vi "Post_Pro_Results_Hierarchy.vi"() -> ()   [LabVIEW 2010]
uses:
  Anemometry Sub Vis/Controls/Setup.ctl
panel:
  out "Error":string
  out "Unfound Files":i32
  out "Processed Files":i32
  in  "Select Plug Ins":bool
  out "Results files Processed":i32(slide) scale=0.0..1.0
  in  "stop":bool
  out "Files To Process":path[](array[path])
  in  "Post processed Results folder":path
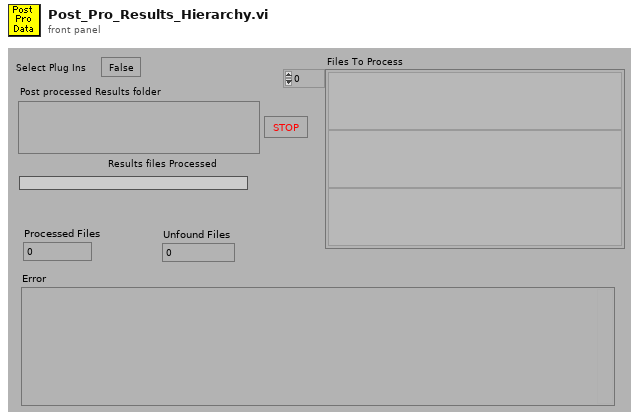
[diagram p1: front panel]
types:
  T1 = typedef "Setup.ctl" = enum16{"Run Program", "Show Setup", "Save Current Setup", "Setup Front Panel"}
  T2 = enum32{"existing file", "new file", "new or existing file", "existing dir", "new dir", "new or existing dir", "existing file (use LLBs)", "new file (use LLBs)", "new or existing file (use LLBs)", "new or existing file or directory (use LLBs)"}
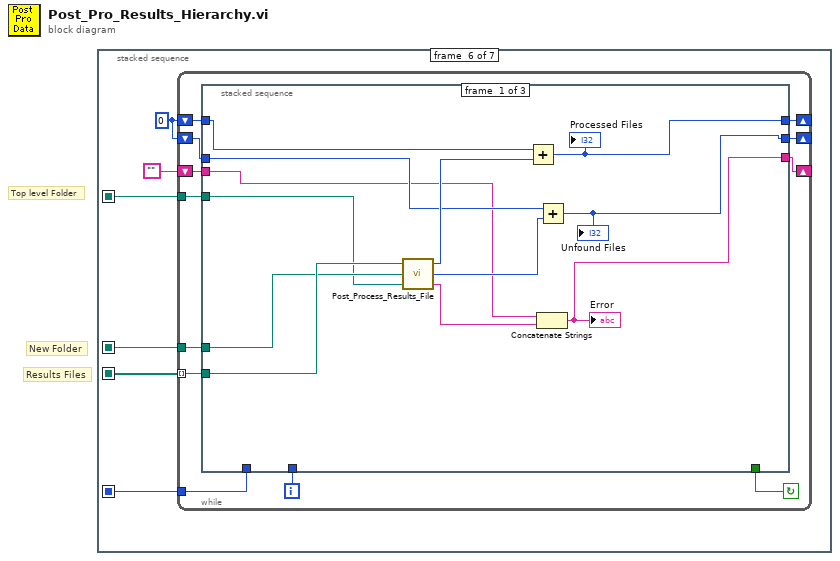
[diagram p0: block diagram]
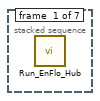
[diagram p2: hidden frame]
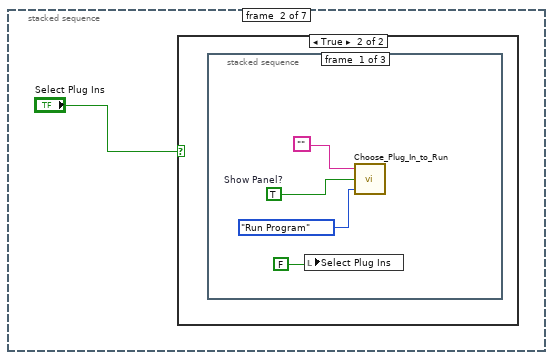
[diagram p3: hidden frame]
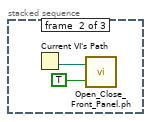
[diagram p5: hidden frame]
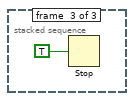
[diagram p6: hidden frame]
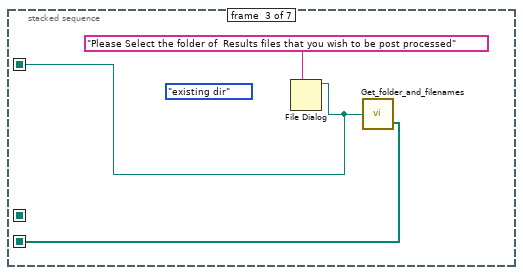
[diagram p7: hidden frame]
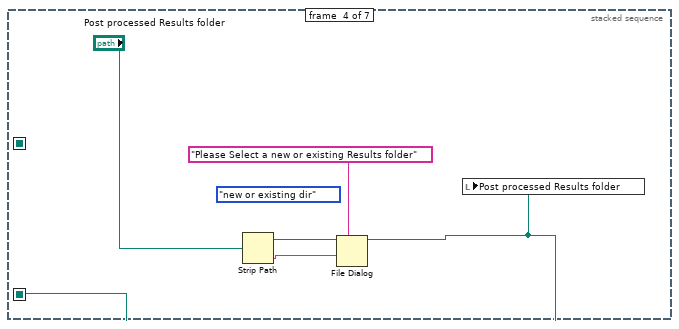
[diagram p8: hidden frame]
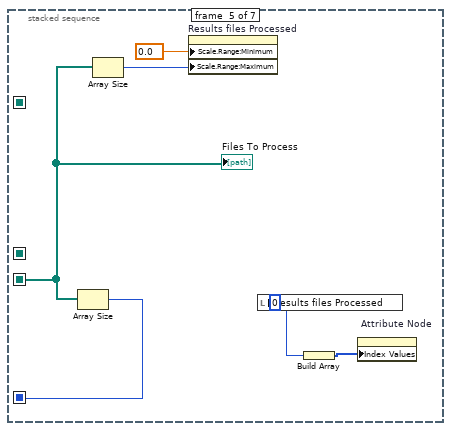
[diagram p9: hidden frame]
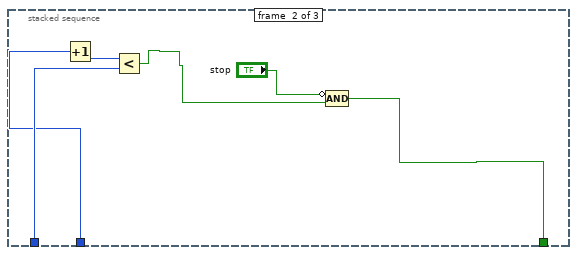
[diagram p10: hidden frame]
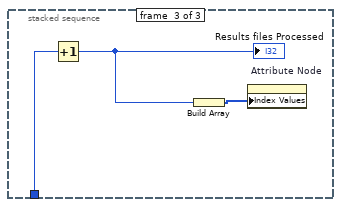
[diagram p11: hidden frame]
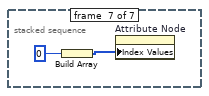
[diagram p12: hidden frame]
diagram:
  # "Top level Folder"
  # "New Folder"
  # "Results Files"
  n1 = stacked-sequence {
    seq-local: [_ _ w9 _ _ _ _] -> [_ _ _ _ _ w25 _]
    seq-local: [_ _ _ _ w22 _ _] -> [_ _ _ _ _ w28 _]
    seq-local: [_ _ _ w16 _ _ _] -> [_ _ _ _ _ w26 _]
    seq-local: [_ _ w10 _ _ _ _] -> [_ _ _ _ w17 w27 _]
    frame #0 {
      n2 = call "Run_EnFlo_Hub.vi"() -> ()  [unwired: 8 in]
    }
    frame #1 {
      n3 = case shown="True" "Select Plug Ins" {
        frame False {
        }
        frame True {
          n4 = stacked-sequence {
            frame #0 {
              w5 = TRUE  # Show Panel?
              n5 = local write "Select Plug Ins"(FALSE ("Select Local ADAM Channels")) -> ()
              n6 = call "Choose_Plug_In_to_Run.vi"("setup"=Setup."Run Program", "Show Panel?"=w5, "Setup String In"="") -> ()  [unwired: 1 in, 1 out]
            }
            frame #1 {
              n7 = Current VI's Path() -> (path=w7:path)
              n8 = call "Open_Close_Front_Panel.ph.vi"("Front Panel Window:Open"=TRUE, "VI path"=w7) -> ()  [unwired: 1 in, 1 out]
            }
            frame #2 {
              n9 = Stop(stop? (T)=TRUE) -> ()
            }
          }
        }
      }
    }
    frame #2 {
      (unwired) T2."existing dir" ("select mode (2)")
      n10 = File Dialog(7:"Please Select the folder of  Results files that you wish to be post processed" ("prompt")) -> (3:w9:path)  [unwired: 6 in, 3 out]
      n11 = call "Get_folder_and_filenames.vi"("file path (dialog if empty)"=w9) -> ("Files"=w10:path[])  [unwired: 1 out]
    }
    frame #3 {
      (unwired) T2."new or existing dir" ("select mode (2)")
      n12 = Strip Path(path="Post processed Results folder") -> (stripped path=w13:path, name=w12:string)
      n13 = File Dialog(7:"Please Select a new or existing Results folder" ("prompt"), 9:w12, 11:w13) -> (3:w16:path)  [unwired: 4 in, 3 out]
      n14 = local write "Post processed Results folder"(w16) -> ()
    }
    frame #4 {
      w18 = 0 ("Files Processed")
      n15 = Array Size(array=w17) -> (size(s)=w22:i32)
      n16 = Array Size(array=w17) -> (size(s)=w20:i32)
      n17 = property on="Results files Processed" class="Slide (strict)"("Scale.Range:Minimum"=0.0 ("Write Attribute"), "Scale.Range:Maximum"=w20) -> ()  [unwired: 2 in, 2 out]
      n18 = local write "Results files Processed"(w18) -> ()
      n19 = Build Array(w18) -> (w19:i32[])
      n20 = property on="Attribute Node" class="Arr (strict)"("Index Values"=w19) -> ()  [unwired: 2 in, 2 out]
      "Files To Process" <- w17
    }
    frame #5 {
      w24 = 0
      n21 = while {
        tunnel: w28 -> [w40]
        tunnel: w27 -> [w37] mode=indexing
        tunnel: w26 -> [w36]
        tunnel: w25 -> [w35]
        shift-right: [w33] -> _
        shift-left: w24 -> [w34]
        shift-right: [w31] -> _
        shift-left: w24 -> [w32]
        shift-right: [w30] -> _
        shift-left: "" -> [w29]
        i -> [w39]
        stop <- w38 continue-if-true
        n22 = stacked-sequence {
          tunnel: w40 -> [_ w56 _]
          tunnel: w39 -> [_ w55 w60]
          tunnel: [_ w54 _] -> w38
          tunnel: w37 -> [w52 _ _]
          tunnel: w36 -> [w51 _ _]
          tunnel: w35 -> [w50 _ _]
          tunnel: w34 -> [w49 _ _]
          tunnel: [w47 _ _] -> w33
          tunnel: w32 -> [w45 _ _]
          tunnel: [w44 _ _] -> w31
          tunnel: w29 -> [w43 _ _]
          tunnel: [w41 _ _] -> w30
          frame #0 {
            n23 = call "Post_Process_Results_File.vi"("Top level Folder"=w50, "Post processed Results folder"=w51, "Results File to Post Process"=w52) -> ("Error"=w42:string, "Files not found"=w46:i32, "File Processed"=w48:i32)
            n24 = Add(x=w49, y=w48) -> (x+y=w47:i32)
            "Processed Files" <- w47
            n25 = Concatenate Strings(w43, w42) -> (w41:string)
            "Error" <- w41
            n26 = Add(x=w45, y=w46) -> (x+y=w44:i32)
            "Unfound Files" <- w44
          }
          frame #1 {
            n27 = Increment(x=w55) -> (x+1=w58:i32)
            n28 = Less?(x=w58, y=w56) -> (x < y?=w57:bool)
            n29 = Compound Arithmetic op=AND(invert "stop", w57) -> (w54:bool)
          }
          frame #2 {
            n30 = Increment(x=w60) -> (x+1=w59:i32)
            "Results files Processed" <- w59
            n31 = Build Array(w59) -> (w61:i32[])
            n32 = property on="Attribute Node" class="Arr (strict)"("Index Values"=w61) -> ()  [unwired: 2 in, 2 out]
          }
        }
      }
    }
    frame #6 {
      n33 = Build Array(0) -> (w63:i32[])
      n34 = property on="Attribute Node" class="Arr (strict)"("Index Values"=w63) -> ()  [unwired: 2 in, 2 out]
    }
  }
